vi "folderPathOrDefaultPath.vi"(7 "defaultPath":path, 11 "File Path Control":path) -> (1 "folder":path, 3 "pathOut":path)   [LabVIEW 2020]
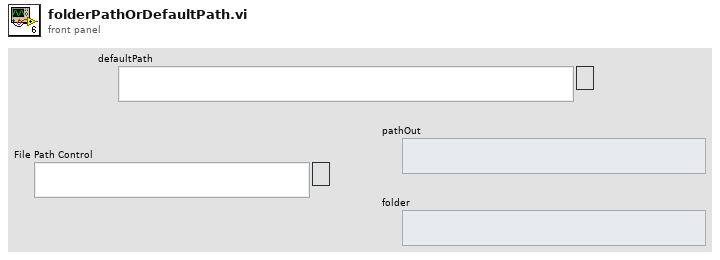
[diagram p1: front panel]
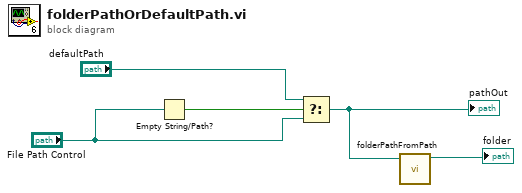
[diagram p0: block diagram]
diagram:
  n1 = Empty String/Path?(string/path="File Path Control") -> (empty?=w5:bool)
  n2 = Select(t="defaultPath", s=w5, f="File Path Control") -> (s? t:f=w1:path)
  "pathOut" <- w1
  n3 = call "folderPathFromPath.vi"("File Path Control"=w1) -> ("stripped path"=→"folder":path)  [unwired: 10 in]
